vi "get_min_max.vi"(8 "error in (no error)":errorcluster, 11 "DAQmxAnalogOut.lvclass in":refnum<class "AnalogOutDL101207DAQmx.lvclass">) -> (0 "error out":errorcluster, 1 "maximum":dbl[unit], 2 "minimum":dbl[unit], 3 "DAQmxAnalogOut.lvclass out":refnum<class "AnalogOutDL101207DAQmx.lvclass">)   [LabVIEW 2010, in "AnalogOutDL101207DAQmx.lvclass"]
uses:
  AnalogOutDL101207DAQmx.lvclass
  AnalogOutDL101207DAQmx.lvclass/AnalogOutDL101207DAQmx.ctl
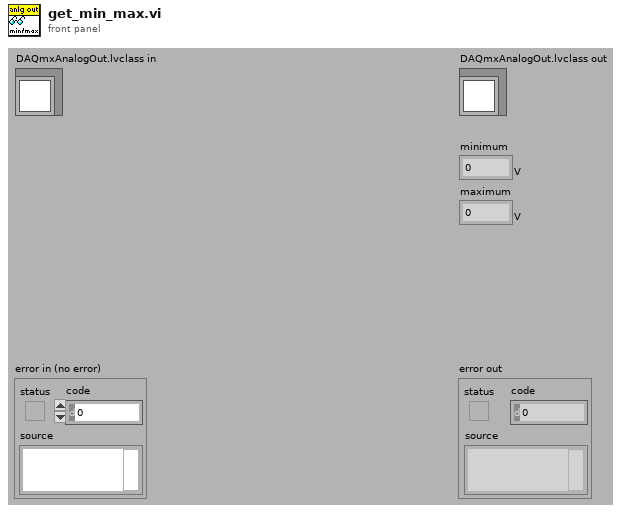
[diagram p1: front panel]
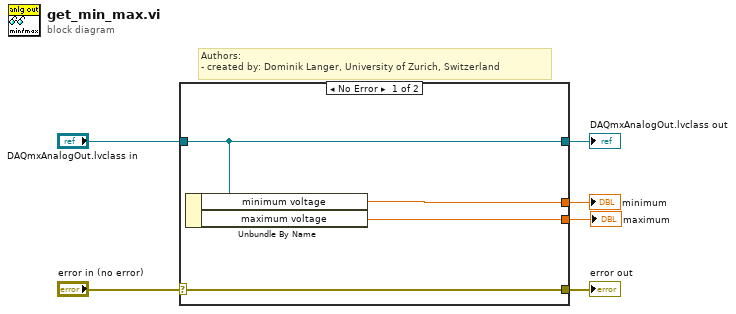
[diagram p0: block diagram]
diagram:
  # "Authors: \n- created by: Dominik Langer, University of Zurich, Switzerland"
  n1 = case shown="No Error" "error in (no error)" {
    selector: "error in (no error)" -> [w10 w11]
    tunnel: [w10 w11] -> w5
    tunnel: [w9 w12] -> w3
    tunnel: "DAQmxAnalogOut.lvclass in" -> [w9 w12]
    tunnel: [w8 _] -> w2
    tunnel: [w7 _] -> w1
    frame No Error {
      n2 = Unbundle By Name(w9) -> ("minimum voltage"=w8:dbl[unit], "maximum voltage"=w7:dbl[unit])
    }
    frame Error {
    }
  }
  "error out" <- w5
  "DAQmxAnalogOut.lvclass out" <- w3
  "minimum" <- w2
  "maximum" <- w1
